vi "Read cassete code.vi"(8 "error in":errorcluster, 10 "Start portBit":i32, 11 "task in":i32) -> (0 "error out":errorcluster, 2 "Casset Code":bool[](array[boolean]), 3 "task out":i32)   [LabVIEW 2023]
uses:
  DO_Reley/DO_Relay.lvlib
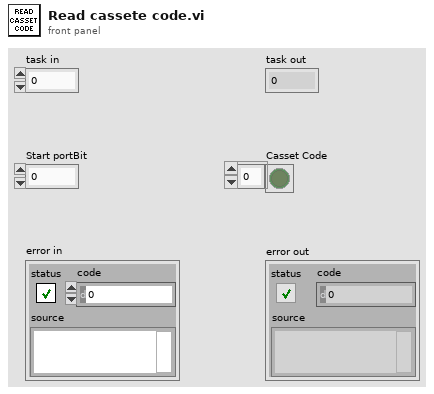
[diagram p1: front panel]
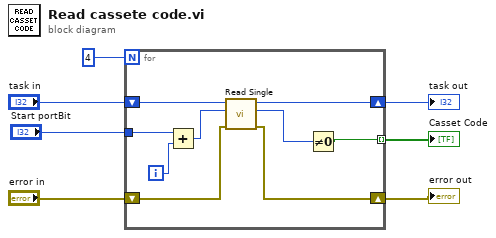
[diagram p0: block diagram]
diagram:
  n1 = for {
    N: 4 -> [_]
    shift-right: [w10] -> w3
    shift-left: "task in" -> [w16]
    tunnel: "Start portBit" -> [w15]
    shift-right: [w11] -> w2
    shift-left: "error in" -> [w12]
    tunnel: [w8] -> w4 mode=indexing
    i -> [w14]
    n2 = Add(x=w15, y=w14) -> (x+y=w13:i32)
    n3 = call "Read Single.vi"("error in"=w12, "portBit"=w13, "task in"=w16) -> ("error out"=w11:errorcluster, "data"=w9:u8, "task out"=w10:i32)  [unwired: 6 in]
    n4 = Not Equal To 0?(x=w9) -> (x != 0?=w8:bool)
  }
  "Casset Code" <- w4
  "task out" <- w3
  "error out" <- w2
